vi "WSVCAP SHL Host TL I2C Read - Single Device.vi"(0 "Bytes to Read (1-4)":u8=4 min=1 max=4 step=1, 3 "FPGA":T1, 5 "Sub Address [U8]":u8=191 format="%.0x", 11 "error in":errorcluster, 12 "DUT":T3, 13 "Device":T2, 14 "Log (T)":bool=TRUE) -> (4 "Device Data":u8[](array[numeric]) format="%.0x", 15 "error out":errorcluster)   [LabVIEW 2012]
uses:
  Type Defs/WSVCAP SHL DUT Number Enum.ctl
  Type Defs/WSVCAP SHL I2C Device Enum.ctl
  Type Defs/WSVCAP SHL I2C FPGA Enum.ctl
panel:
  out "C3:1-36 Read Data [U8]":u8[][](array[numeric]) format="%.0x"
  out "Socket Mask Set [U64]":u64[](array[numeric]) format="%012x"
  out "C2:1-36 Read Data [U8]":u8[][](array[numeric]) format="%.0x"
  out "C1:1-36 Read Data [U8]":u8[][](array[numeric]) format="%.0x"
  out "Data Headers":u8[](array[numeric])=[1, 2, 3, 4, 5, 6, 7, 8, 9, 10, 11, 12, 12, 14, 15, 16, 17, 18, 19, 20, 21, 22, 23, 24, 25, 26, 27, 28, 29, 30, 31, 32, 33, 34, 35, 36]
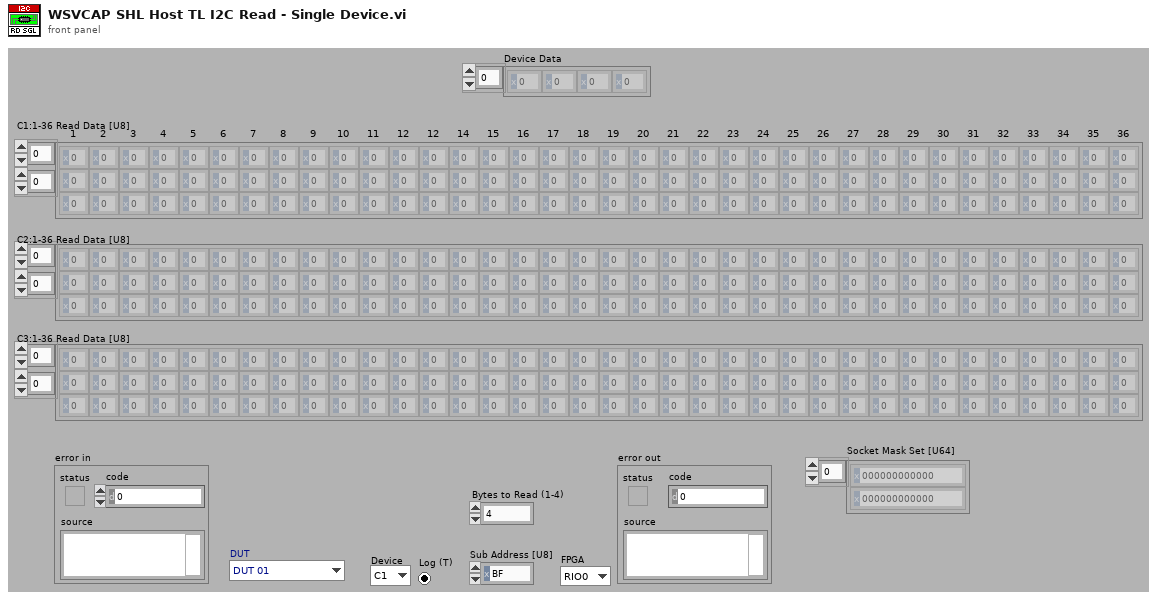
[diagram p1: front panel]
types:
  T1 = typedef "WSVCAP SHL I2C FPGA Enum.ctl" = enum16{"RIO0", "RIO1"}
  T2 = typedef "WSVCAP SHL I2C Device Enum.ctl" = enum16{"C1", "C2", "C3"}
  T3 = typedef "WSVCAP SHL DUT Number Enum.ctl" = enum16{"DUT 01", "DUT 02", "DUT 03", "DUT 04", "DUT 05", "DUT 06", "DUT 07", "DUT 08", "DUT 09", "DUT 10", "DUT 11", "DUT 12", "DUT 13", "DUT 14", "DUT 15", "DUT 16", "DUT 17", "DUT 18", "DUT 19", "DUT 20", "DUT 21", "DUT 22", "DUT 23", "DUT 24", "DUT 25", "DUT 26", "DUT 27", "DUT 28", "DUT 29", "DUT 30", "DUT 31", "DUT 32", "DUT 33", "DUT 34", "DUT 35", "DUT 36"}
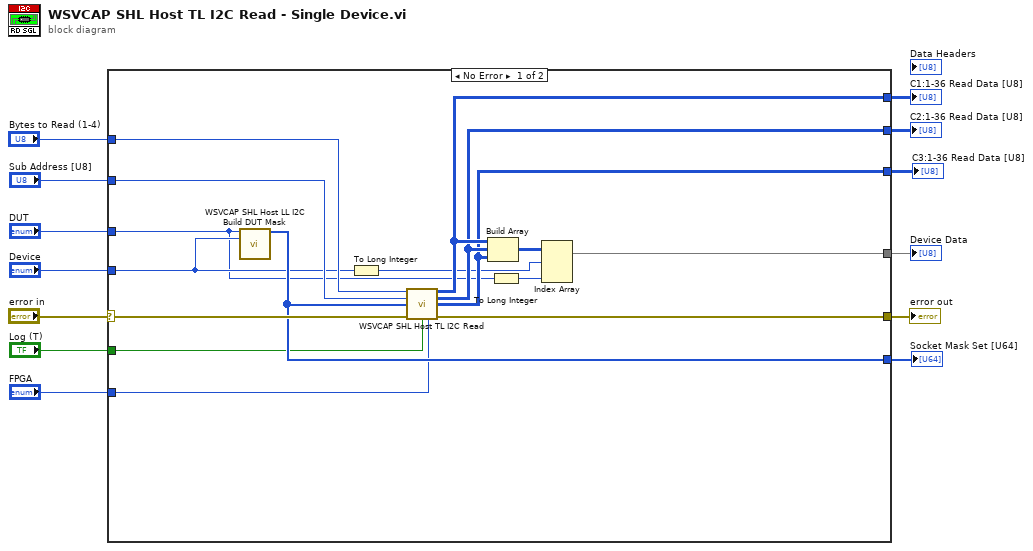
[diagram p0: block diagram]
diagram:
  n1 = case shown="No Error" "error in" {
    selector: "error in" -> [w28 w30]
    tunnel: [w29 w30] -> w13
    tunnel: "Bytes to Read (1-4)" -> [w27 _]
    tunnel: "Sub Address [U8]" -> [w26 _]
    tunnel: "DUT" -> [w15 _]
    tunnel: [w25 _] -> w8
    tunnel: "Device" -> [w17 _]
    tunnel: [w22 _] -> w6
    tunnel: [w21 _] -> w5
    tunnel: [w24 _] -> w4
    tunnel: "Log (T)" -> [w23 _]
    tunnel: [w20 _] -> w2
    tunnel: "FPGA" -> [w14 _]
    frame No Error {
      n2 = call "WSVCAP SHL Host LL I2C Build DUT Mask.vi"("DUT"=w15, "Device"=w17) -> ("Socket Mask Set [U64]"=w25:u64[])  [unwired: 12 in, 1 out]
      n3 = To Long Integer(number=w17) -> (32bit integer=w16:i32)
      n4 = call "WSVCAP SHL Host TL I2C Read.vi"("Bytes to Read"=w27, "Sub Address [U8]"=w26, "Socket Mask Set [U64]"=w25, "error in"=w28, "Log (T)"=w23, "FPGA"=w14) -> ("C1 Read Data Out"=w22:u8[][], "C2 Read Data Out"=w21:u8[][], "C3 Read Data Out"=w20:u8[][], "error out"=w29:errorcluster)  [unwired: 6 in]
      n5 = Build Array(w22, w21, w20) -> (w19:u8[][][])
      n6 = To Long Integer(number=w15) -> (32bit integer=w18:i32)
      n7 = Index Array(array=w19, index (dim 0)=w16, index (dim 2)=w18) -> (element=w24:u8[])  [unwired: 1 in]
    }
    frame Error {
    }
  }
  "error out" <- w13
  "Socket Mask Set [U64]" <- w8
  "C1:1-36 Read Data [U8]" <- w6
  "C2:1-36 Read Data [U8]" <- w5
  "Device Data" <- w4
  "C3:1-36 Read Data [U8]" <- w2
